vi "get_map.vi"(4 "error in":errorcluster={"status"=FALSE, "code"=0, "source"="Event Code: 0\r\nweather configured to \"Default\"\r\n-----------------------------------\nEvent Code: 0\r\n\r\n-----------------------------------\n"}, 6 "message":string="{\t\t\"gis_anchor\": {\n\t\t\t\"x\": 40.410262,\n\t\t\t\"y\": -79.948172,\n\t\t\t\"z\": 1\n\t\t},\n\t\t\"orientation\": -16.5,\n\t\t\"point_delta\": 100.0,\n\t\t\"coordinates\": \"world\",\n   \"format\": \"point_array\"\n}\n", 7 "simx in":T1={"Config"={"Trajectory"={"Number of frames"=0, "Frame number"=0, "Trajectory"=""}, "Weather"={"id"=""}}, "Connections"={"Simulator Connection"=refnum, "server_ip"="127.0.0.1", "Port"=0, "Sensor connections"=[]}, "Map"={"lanes"={"x"=[], "y"=[], "z"=[]}, "StartPosition"={"start_points"={"locations"=[], "rotations"=[], "type"=[]}, "StartRotation"=[], "StartLocation"=[]}, "Draw Map Size"={"Width"=0, "Height"=0}, "DrawArea"={"min_Y"=0.0, "min_X"=0.0, "Scale X"=0.0, "Scale Y"=0.0}, "Map"=bytes[0], "Map Geojson"=""}}) -> (0 "error out":errorcluster, 3 "simx out":T1={"Config"={"Trajectory"={"Number of frames"=0, "Frame number"=0, "Trajectory"=""}, "Weather"={"id"=""}}, "Connections"={"Simulator Connection"=refnum, "server_ip"="127.0.0.1", "Port"=0, "Sensor connections"=[]}, "Map"={"lanes"={"x"=[], "y"=[], "z"=[]}, "StartPosition"={"start_points"={"locations"=[], "rotations"=[], "type"=[]}, "StartRotation"=[], "StartLocation"=[]}, "Draw Map Size"={"Width"=0, "Height"=0}, "DrawArea"={"min_Y"=0.0, "min_X"=0.0, "Scale X"=0.0, "Scale Y"=0.0}, "Map"=bytes[0], "Map Geojson"=""}})   [LabVIEW 2019]
doc: "Send the GetMap command to obtain the map data in GeoJSON or array format."
uses:
  controls/simx_connection.ctl
  controls/config.ctl
  controls/trajectory.ctl
  controls/weather.ctl
  controls/connections.ctl
  controls/start_points.ctl
  <vilib>/Utility/miscctls.llb/LVBoundsTypeDef.ctl
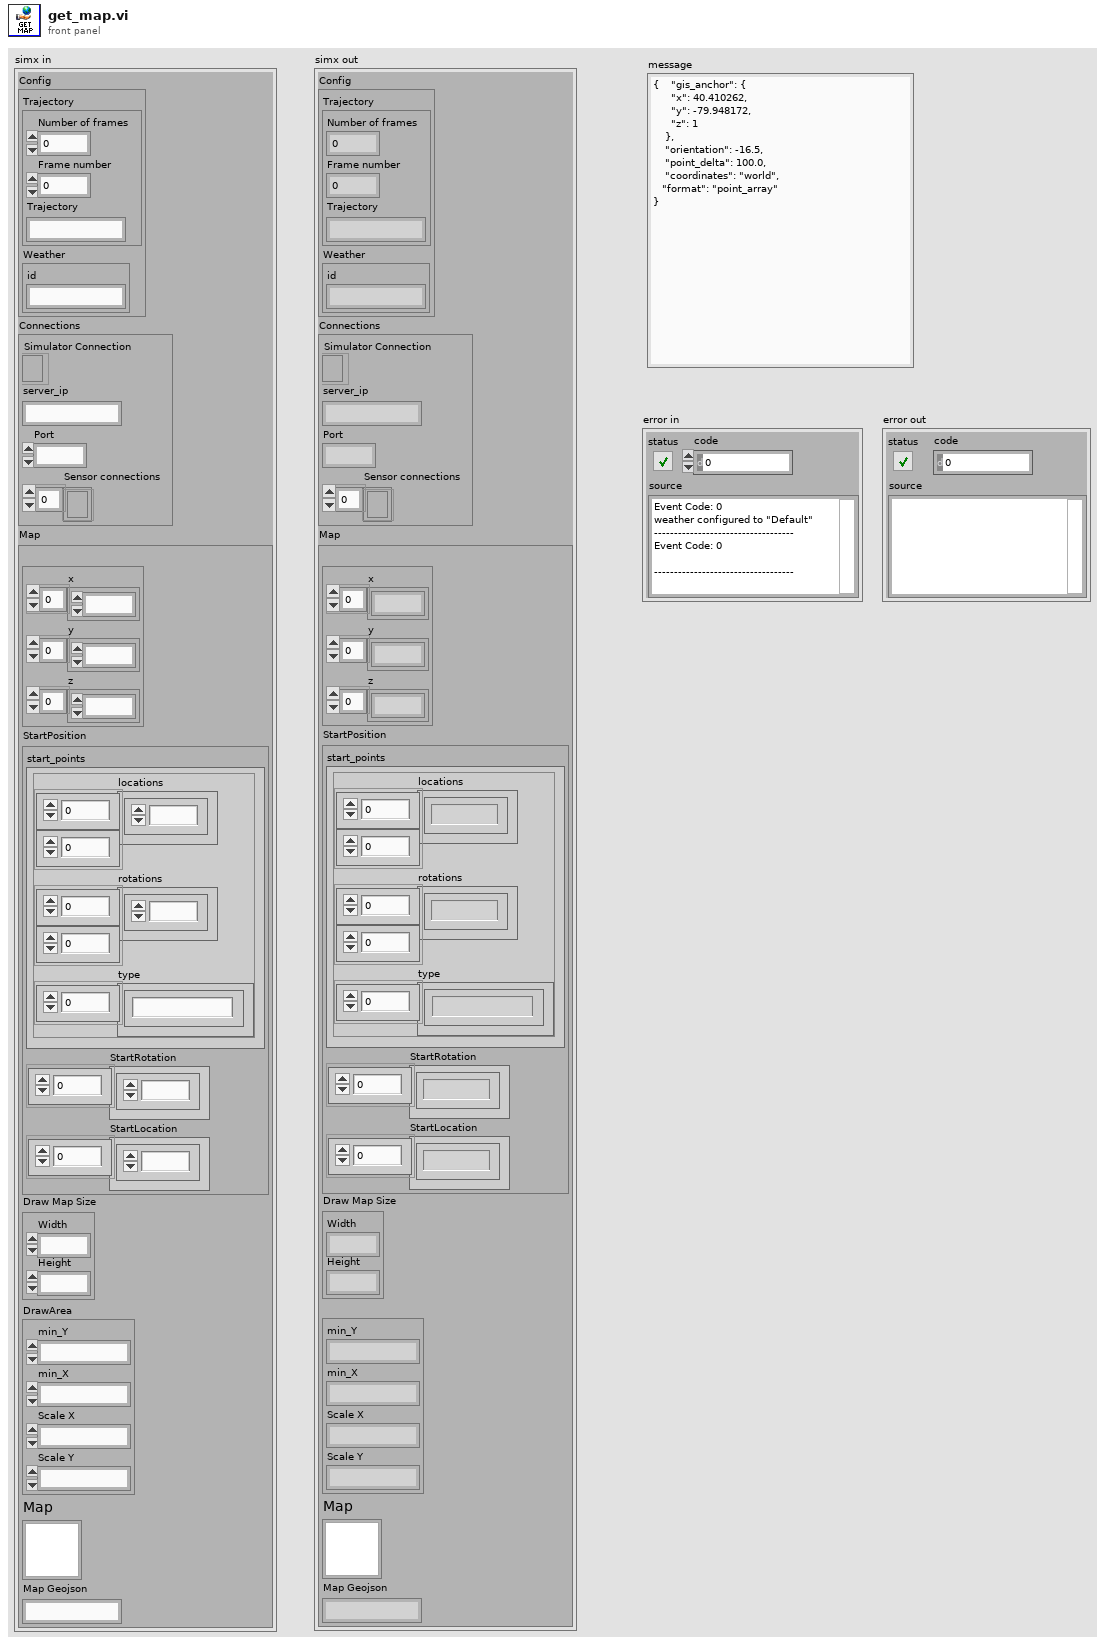
[diagram p1: front panel]
types:
  T1 = typedef "simx_connection.ctl" = cluster{"Config":T2, "Connections":T5, "Map":cluster{"lanes":cluster{"x":dbl[], "y":dbl[], "z":dbl[]}, "StartPosition":cluster{"start_points":T6, "StartRotation":dbl[], "StartLocation":dbl[]}, "Draw Map Size":T7, "DrawArea":cluster{"min_Y":dbl, "min_X":dbl, "Scale X":dbl, "Scale Y":dbl}, "Map":picture, "Map Geojson":string}}
  T2 = typedef "config.ctl" = cluster{"Trajectory":T3, "Weather":T4}
  T3 = typedef "trajectory.ctl" = cluster{"Number of frames":i32, "Frame number":i32, "Trajectory":string}
  T4 = typedef "weather.ctl" = cluster{"id":string}
  T5 = typedef "connections.ctl" = cluster{"Simulator Connection":refnum<k5>, "server_ip":string, "Port":i32, "Sensor connections":refnum<k5>[]}
  T6 = typedef "start_points.ctl" = cluster{"locations":dbl[][], "rotations":dbl[][], "type":string[]}
  T7 = typedef "LVBoundsTypeDef.ctl" = cluster{"Width":u32, "Height":u32}
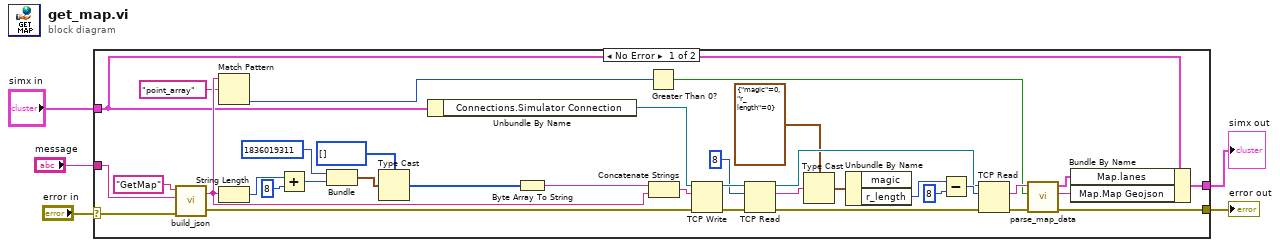
[diagram p0: block diagram]
diagram:
  n1 = case shown="No Error" "error in" {
    selector: "error in" -> [w38 w42]
    tunnel: "simx in" -> [w36 w43]
    tunnel: [w35 w43] -> w3
    tunnel: [w37 w42] -> w2
    tunnel: "message" -> [w34 _]
    frame No Error {
      n2 = call "build_json.vi"("error in"=w38, "Message"=w34, "Command_ID"="GetMap") -> ("error out"=w40:errorcluster, "JSON Out"=w39:string)  [unwired: 1 in]
      n3 = Match Pattern(string=w39, regular expression="point_array") -> (offset past match=w7:i32)  [unwired: 1 in, 3 out]
      n4 = String Length(string=w39) -> (length=w14:i32)
      n5 = Add(x=w14, y=u32 8) -> (x+y=w25:u32)
      n6 = Bundle(u32 1836019311, w25) -> (w30:cluster{u32, u32})  [unwired: 1 in]
      n7 = Type Cast(type=u8[] [], x=w30) -> (*(type *) &x=w28:u8[])
      n8 = Unbundle By Name(w36) -> ("Connections.Simulator Connection"=w33:refnum<k5>)
      n9 = Byte Array To String(unsigned byte array=w28) -> (string=w24:string)
      n10 = Greater Than 0?(x=w7) -> (x > 0?=w6:bool)
      n11 = Concatenate Strings(w24, w39) -> (w13:string)
      n12 = TCP Write(connection ID=w33, data in=w13, error in (no error)=w40) -> (connection ID out=w31:refnum<k5>, error out=w32:errorcluster)  [unwired: 1 in, 1 out]
      n13 = TCP Read(connection ID=w31, bytes to read=8, error in (no error)=w32) -> (connection ID out=w18:refnum<k5>, data out=w23:string, error out=w19:errorcluster)  [unwired: 2 in]
      n14 = Type Cast(type=cluster{"magic":u32, "r_length":u32} {"magic"=0, "r_length"=0}, x=w23) -> (*(type *) &x=w22:cluster{"magic":u32, "r_length":u32})
      n15 = Unbundle By Name(w22) -> ("r_length"=w20:u32)  [unwired: 1 out]
      n16 = Subtract(x=w20, y=u32 8) -> (x-y=w21:u32)
      n17 = TCP Read(connection ID=w18, bytes to read=w21, error in (no error)=w19) -> (data out=w11:string, error out=w12:errorcluster)  [unwired: 2 in, 1 out]
      n18 = call "parse_map_data.vi"("error in"=w12, "Array?"=w6, "Map"=w11) -> ("error out"=w37:errorcluster, "Map Geojson"=w9:string, "Lanes"=w10:cluster{"x":dbl[], "y":dbl[], "z":dbl[]})  [unwired: 2 in]
      n19 = Bundle By Name(cluster=w36, "Map.lanes"=w10, "Map.Map Geojson"=w9) -> (w35:T1)
    }
    frame Error {
    }
  }
  "simx out" <- w3
  "error out" <- w2
